vi "Find EXP Interval.vi"(8 "error in (no error)":errorcluster, 9 "Data":variant, 11 "Scan Data Process in":T1) -> (0 "error out":errorcluster, 1 "Start Time":timestamp, 2 "Trigger?":bool, 3 "Scan Data Process out":T1)   [LabVIEW 2015, in "Exposure Process.lvlib"]
uses:
  Exposure Process.lvlib
  Control_Scan Data Process.ctl
  <vilib>/addons/PointValueMap/controls/PointMap.ctl
  Control_EXP Information.ctl
  Control_File Save Setup.ctl
  Control_Enable and Path.ctl
  Control_ICM Export Setting.ctl
  <vilib>/addons/PointValueMap/PointValueMap.lvlib
panel:
  out "Waveform Graph":waveform(dbl)(graph)
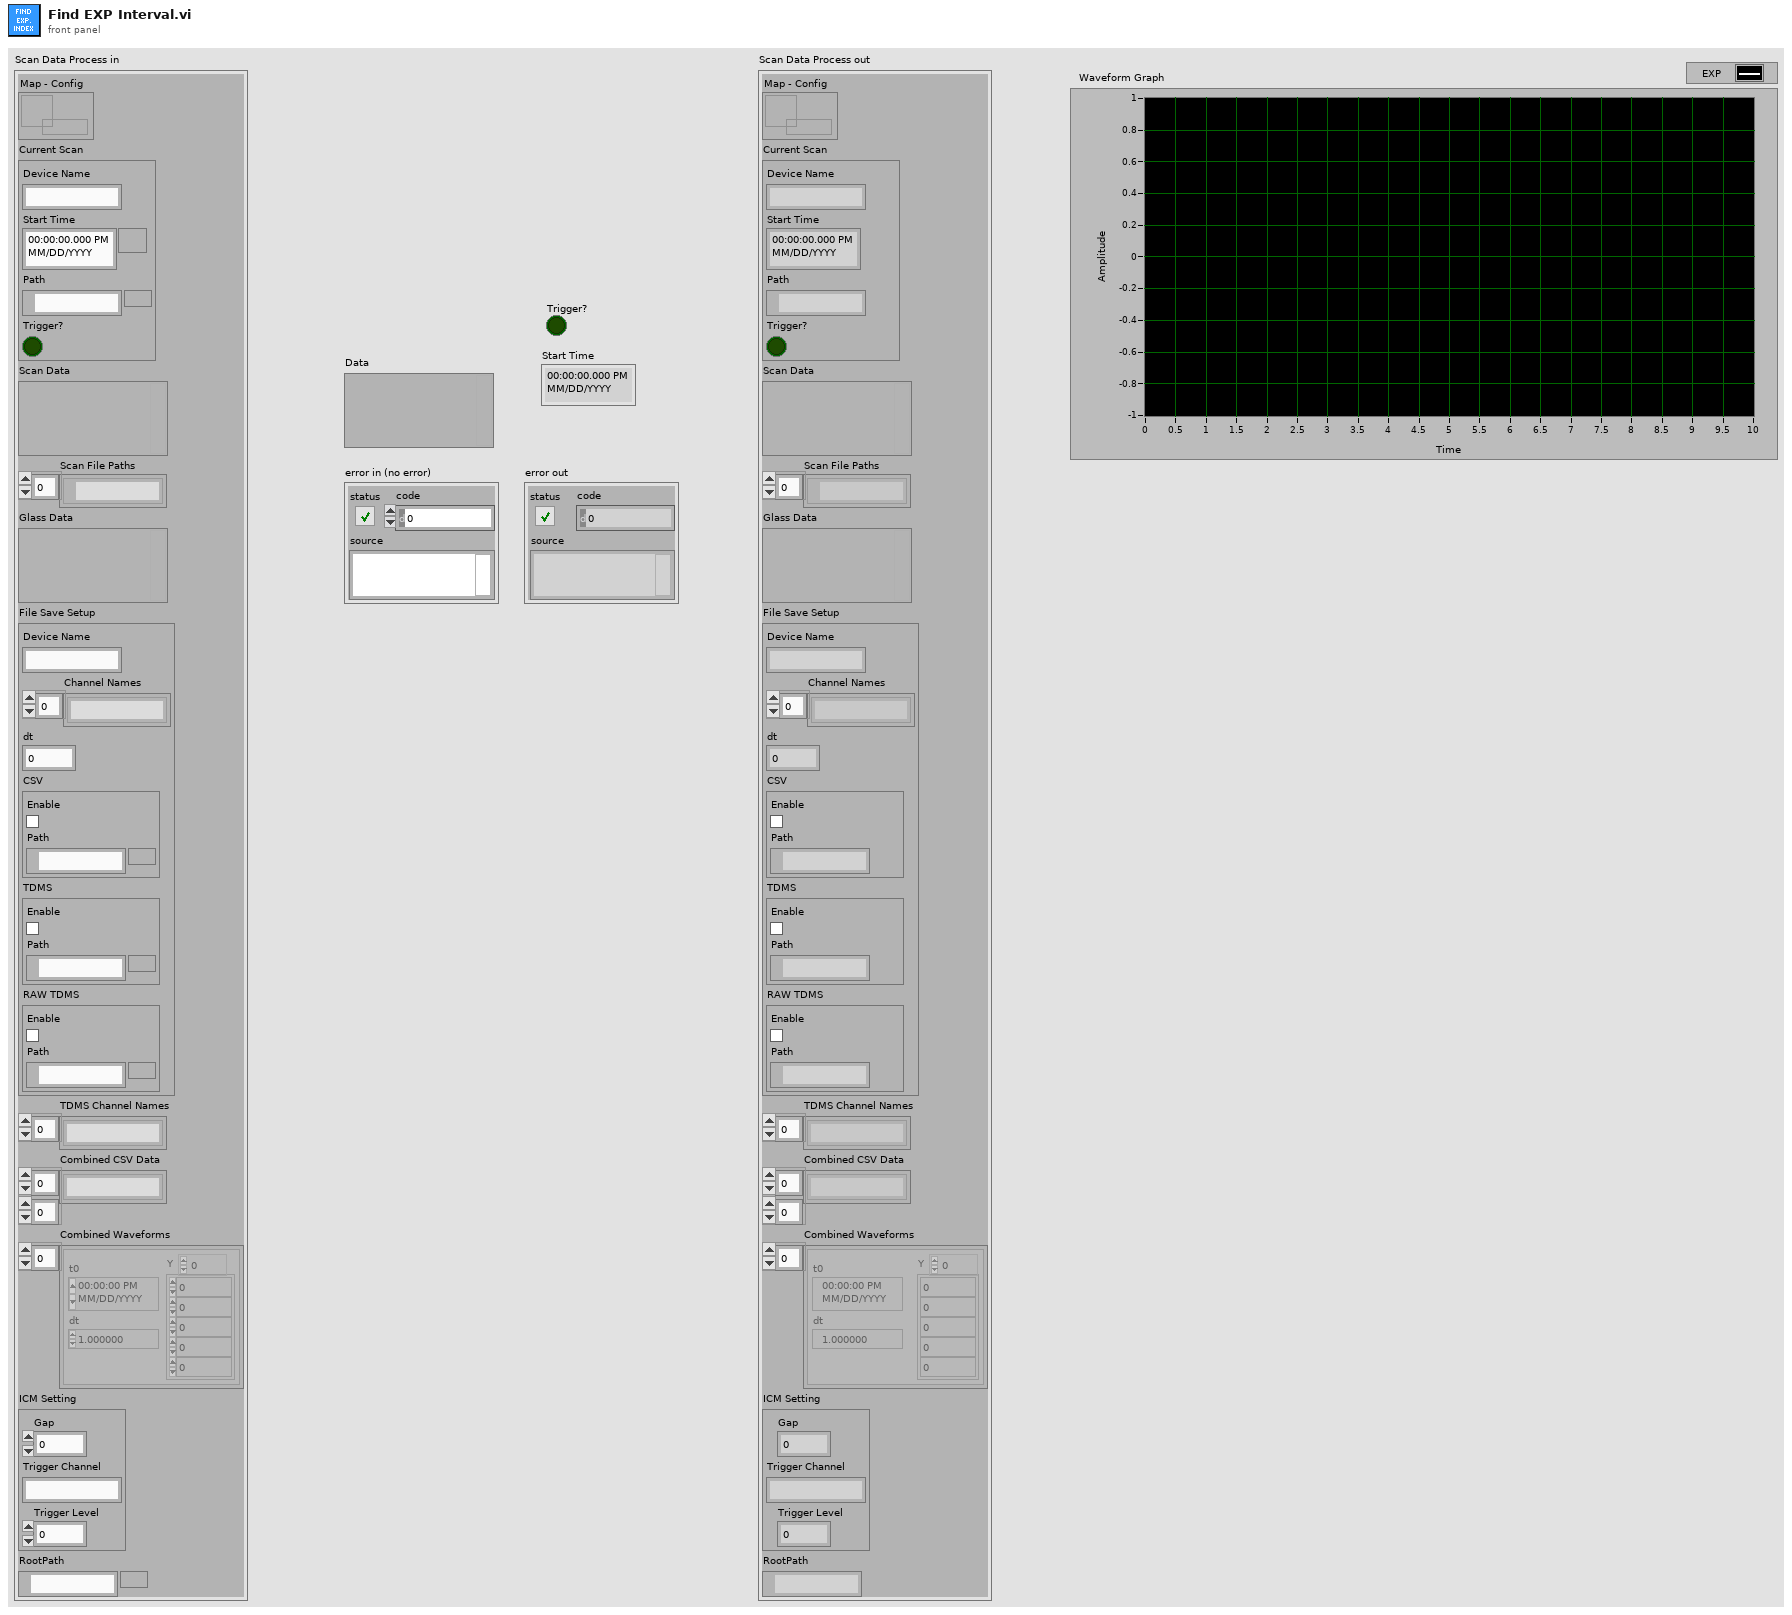
[diagram p1: front panel]
types:
  T1 = typedef "Exposure Process.lvlib/Control_Scan Data Process.ctl" = cluster{"Map - Config":T2, "Current Scan":T3, "Scan Data":variant, "Scan File Paths":path[], "Glass Data":variant, "File Save Setup":T4, "TDMS Channel Names":string[], "Combined CSV Data":string[][], "Combined Waveforms":waveform(dbl)[], "ICM Setting":T6, "RootPath":path}
  T2 = typedef "PointValueMap.lvlib/PointMap.ctl" = refnum<data-value>
  T3 = typedef "Exposure Process.lvlib/Control_EXP Information.ctl" = cluster{"Device Name":string, "Start Time":timestamp, "Path":path, "Trigger?":bool}
  T4 = typedef "Exposure Process.lvlib/Control_File Save Setup.ctl" = cluster{"Device Name":string, "Channel Names":string[], "dt":dbl, "CSV":T5, "TDMS":T5, "RAW TDMS":T5}
  T5 = typedef "Exposure Process.lvlib/Control_Enable and Path.ctl" = cluster{"Enable":bool, "Path":path}
  T6 = typedef "Exposure Process.lvlib/Control_ICM Export Setting.ctl" = cluster{"Gap":dbl, "Trigger Channel":string, "Trigger Level":dbl}
  T7 = typedef "Exposure Process.lvlib/Control_Start-End-Trigger.ctl" = cluster{"start_index":i64, "end_index":i64, "trigger_count":i64}
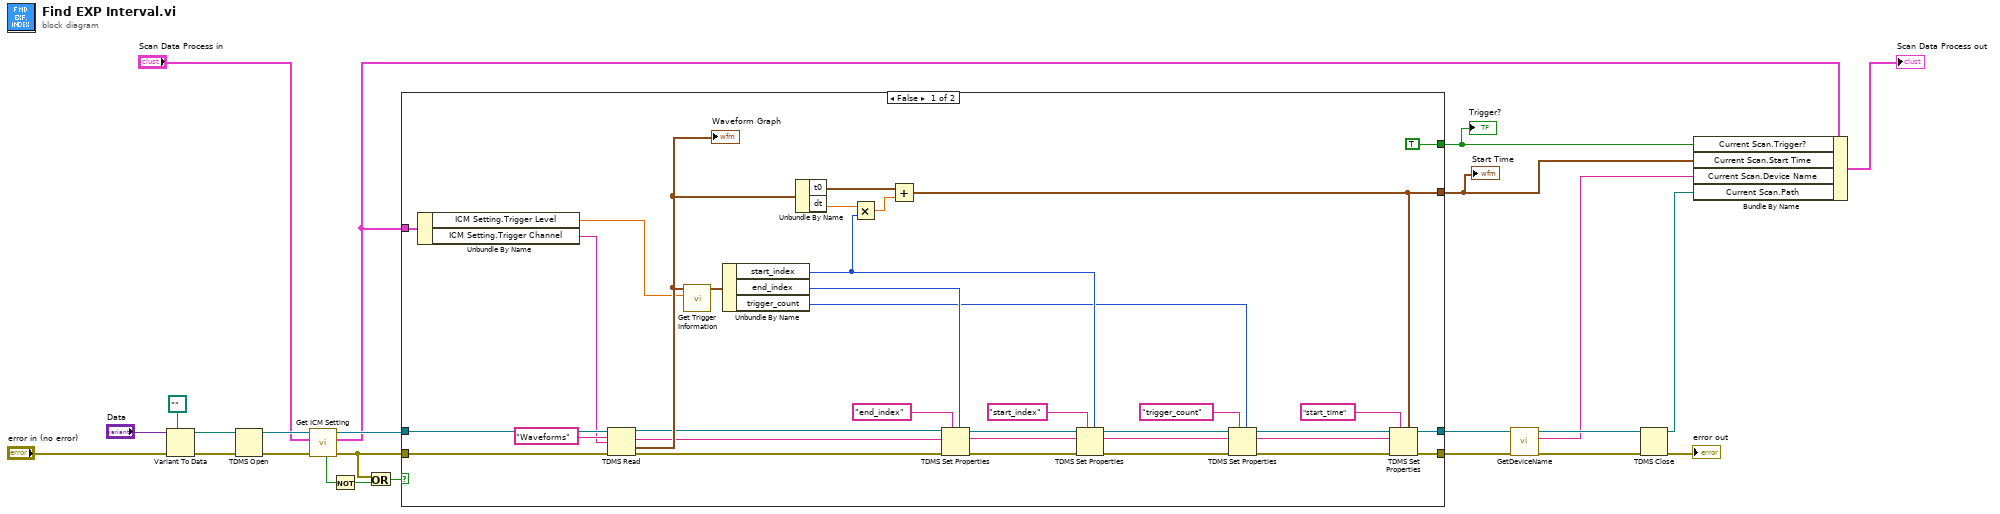
[diagram p0: block diagram]
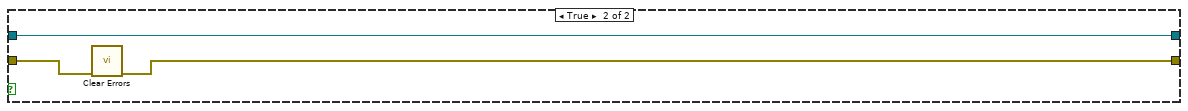
[diagram p2: hidden frame]
diagram:
  n1 = Variant To Data(error in="error in (no error)", type=path "", Variant="Data") -> (data=w22:path, error out=w21:errorcluster)
  n2 = TDMS Open(8:w21, 11:w22) -> (0:w13:errorcluster, 3:w14:refnum<k34>)  [unwired: 5 in]
  n3 = call "Get ICM Setting.vi"("error in (no error)"=w13, "Scan Data Process in"="Scan Data Process in", "tdms file"=w14) -> ("error out"=w8:errorcluster, "Scan Data Process out"=w10:T1, "tdms file out"=w12:refnum<k34>, "Vaild?"=w7:bool)  [unwired: 5 in]
  n4 = Not(x=w7) -> (.not. x?=w6:bool)
  n5 = Or(x=w8, y=w6) -> (x .or. y?=w9:bool)
  n6 = case shown="False" w9 {
    tunnel: w12 -> [w34 w61]
    tunnel: [w45 w61] -> w5
    tunnel: [w41 w60] -> w4
    tunnel: [w40 _] -> w17
    tunnel: [TRUE _] -> w18
    tunnel: w10 -> [w32 _]
    tunnel: w8 -> [w25 w59]
    frame False {
      n7 = Unbundle By Name(w32) -> ("ICM Setting.Trigger Level"=w31:dbl, "ICM Setting.Trigger Channel"=w29:string)
      n8 = TDMS Read(0:w34, 5:"Waveforms" ("group name in"), 7:w29, 11:w25) -> (4:w28:refnum<k34>, 6:w26:string, 10:w33:waveform(dbl), 15:w27:errorcluster)  [unwired: 4 in, 2 out]
      "Waveform Graph" <- w33
      n9 = call "Get Trigger Information.vi"("level"=w31, "Waveform"=w33) -> ("Trigger Information"=w38:T7)  [unwired: 9 in]
      n10 = Unbundle By Name(w38) -> ("start_index"=w37:i64, "end_index"=w36:i64, "trigger_count"=w35:i64)
      n11 = Unbundle By Name(w33) -> ("t0"=w57:timestamp, "dt"=w58:dbl)
      n12 = Multiply(x=w58, y=w37) -> (x*y=w56:dbl)
      n13 = Add(x=w57, y=w56) -> (x+y=w40:timestamp)
      n14 = TDMS Set Properties(5:w36, 7:"end_index", 8:w27, 10:w26, 11:w28) -> (0:w52:errorcluster, 2:w51:string, 3:w53:refnum<k34>)  [unwired: 1 in, 1 out]
      n15 = TDMS Set Properties(5:w37, 7:"start_index", 8:w52, 10:w51, 11:w53) -> (0:w47:errorcluster, 2:w48:string, 3:w49:refnum<k34>)  [unwired: 1 in, 1 out]
      n16 = TDMS Set Properties(5:w35, 7:"trigger_count", 8:w47, 10:w48, 11:w49) -> (0:w42:errorcluster, 2:w43:string, 3:w44:refnum<k34>)  [unwired: 1 in, 1 out]
      n17 = TDMS Set Properties(5:w40, 7:"start_time", 8:w42, 10:w43, 11:w44) -> (0:w41:errorcluster, 3:w45:refnum<k34>)  [unwired: 1 in, 2 out]
    }
    frame True {
      n18 = call <vilib>:"Clear Errors.vi"("error in (no error)"=w59) -> ("error out"=w60:errorcluster)  [unwired: 5 in, 1 out]
    }
  }
  "Start Time" <- w17
  "Trigger?" <- w18
  n19 = call "GetDeviceName.vi"("error in (no error)"=w4, "tdms file"=w5) -> ("error out"=w3:errorcluster, "Device Name"=w1:string, "tdms file out"=w2:refnum<k34>)  [unwired: 7 in]
  n20 = TDMS Close(8:w3, 11:w2) -> (0:→"error out":errorcluster, 3:w16:path)
  n21 = Bundle By Name(cluster=w10, "Current Scan.Trigger?"=w18, "Current Scan.Start Time"=w17, "Current Scan.Device Name"=w1, "Current Scan.Path"=w16) -> (→"Scan Data Process out":T1)
